vi "e.gate ASCII Read Value - CORE.vi"(8 "error in (no error)":errorcluster, 9 "Channel":i32, 11 "e.gate Configuration In":T1) -> (0 "error out":errorcluster, 2 "Value":dbl, 3 "e.gate Configuration Out":T1)   [LabVIEW 2016]
doc: "<B>AMC - Analytik & Messtechnik GmbH Chemnitz</B>\n\nLabVIEW Drivers for e.gate / e.pac series from Gantner Instruments\n\nThis VI reads a value specified by <B>Channel</B> from a device specified by <B>connection ID In</B>."
uses:
  e.gate Configuration.ctl
  e.gate Channel Data.ctl
  e.gate Data Type.ctl
  e.gate Protocol Type.ctl
  e.gate Module  Data.ctl
  e.gateHSP_DLLhandle.ctl
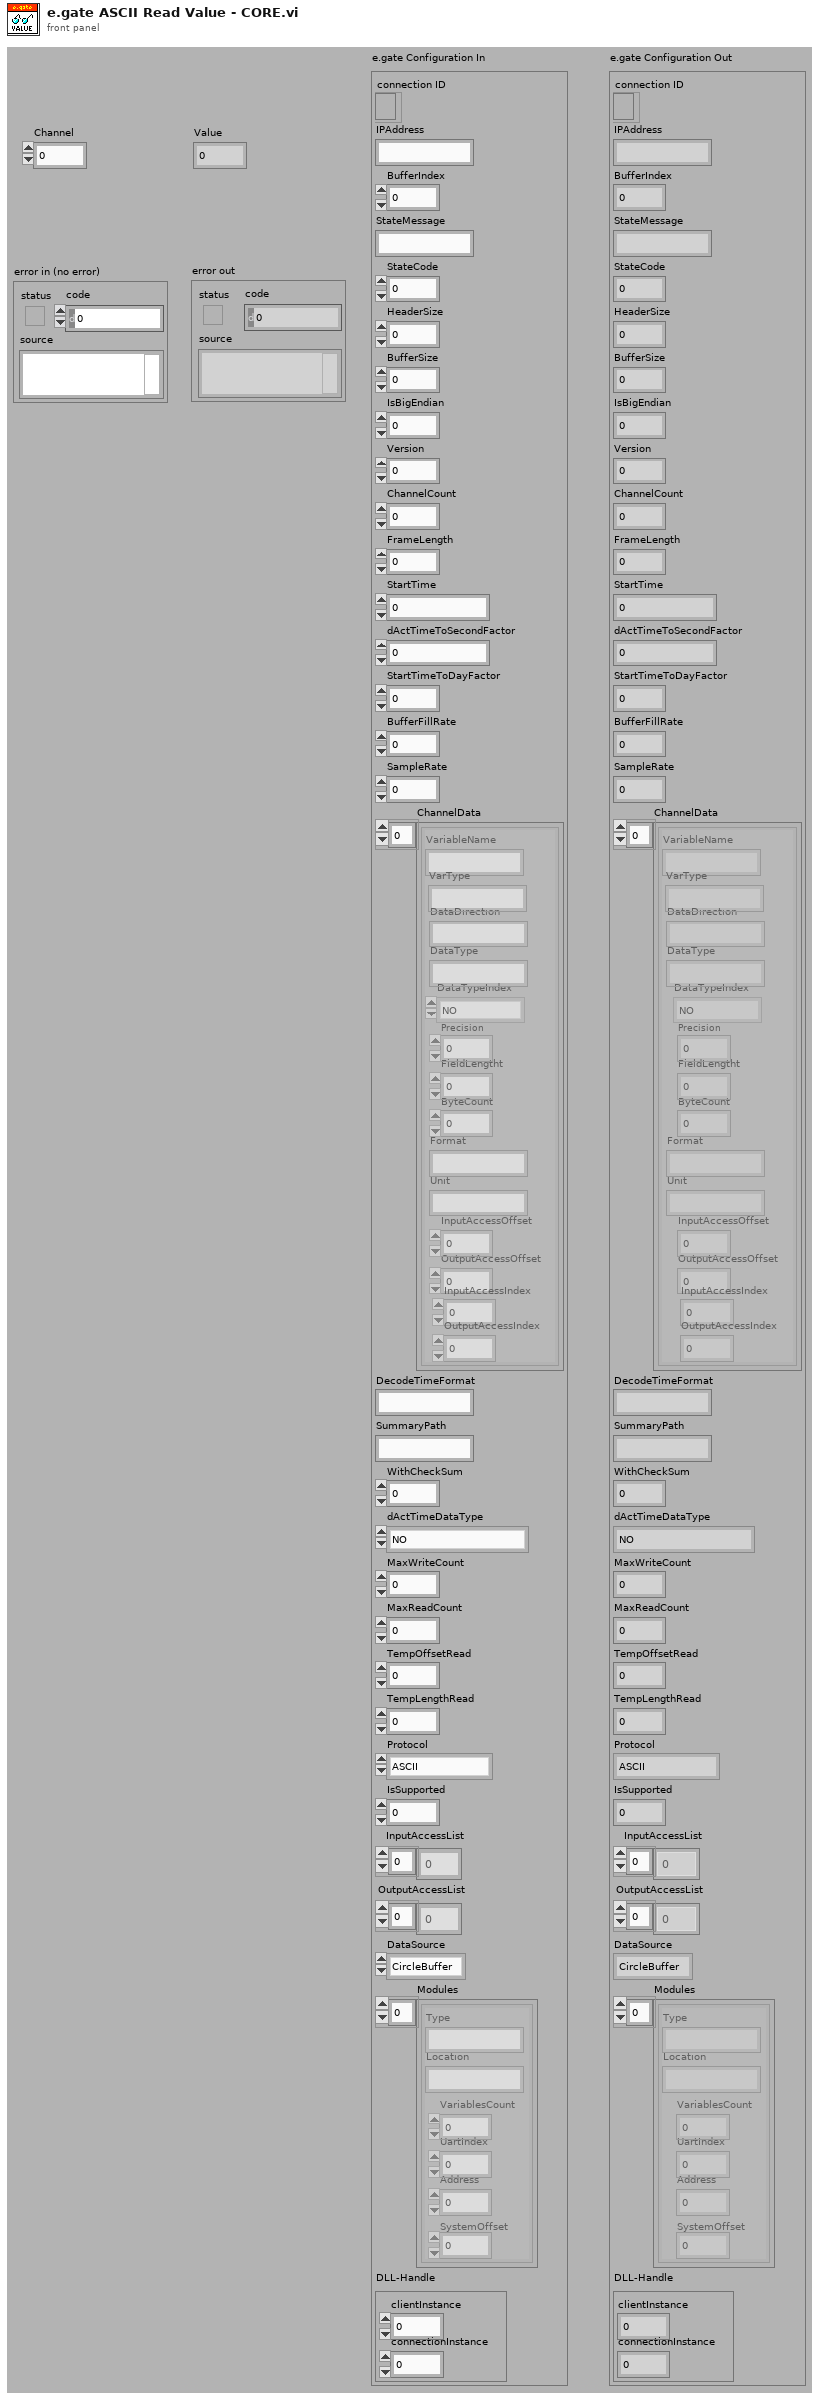
[diagram p1: front panel]
types:
  T1 = typedef "e.gate Configuration.ctl" = cluster{"connection ID":refnum<k5>, "IPAddress":string, "BufferIndex":i32, "StateMessage":string, "StateCode":i8, "HeaderSize":i32, "BufferSize":i32, "IsBigEndian":i32, "Version":i32, "ChannelCount":i32, "FrameLength":i32, "StartTime":dbl, "dActTimeToSecondFactor":dbl, "StartTimeToDayFactor":dbl, "BufferFillRate":dbl, "SampleRate":dbl, "ChannelData":T2[], "DecodeTimeFormat":string, "SummaryPath":string, "WithCheckSum":i32, "dActTimeDataType":T3, "MaxWriteCount":i32, "MaxReadCount":i32, "TempOffsetRead":i32, "TempLengthRead":i32, "Protocol":T4, "IsSupported":i32, "InputAccessList":i32[], "OutputAccessList":i32[], "DataSource":enum16{"CircleBuffer", "test.con Logger", "test.con Archive"}, "Modules":T5[], "DLL-Handle":T6}
  T2 = typedef "e.gate Channel Data.ctl" = cluster{"VariableName":string, "DataDirection":string, "DataType":string, "DataTypeIndex":T3, "Precision":i16, "FieldLengtht":i16, "ByteCount":i32, "Format":string, "Unit":string, "InputAccessOffset":i32, "OutputAccessOffset":i16, "InputAccessIndex":i16, "OutputAccessIndex":i16, "VarType":string}
  T3 = typedef "e.gate Data Type.ctl" = enum16{"NO", "BOOL", "SINT8", "USINT8", "SINT16", "USINT16", "SINT32", "USINT32", "FLOAT", "SET8", "SET16", "SET32", "DOUBLE", "SINT64", "USINT64", "SET64"}
  T4 = typedef "e.gate Protocol Type.ctl" = enum16{"ASCII", "HighspeedPort Online", "HighspeedPort Buffer", "eGateHighspeedPortDLL "}
  T5 = typedef "e.gate Module  Data.ctl" = cluster{"Type":string, "Location":string, "VariablesCount":i16, "UartIndex":i16, "Address":i16, "SystemOffset":i16}
  T6 = typedef "e.gateHSP_DLLhandle.ctl" = cluster{"clientInstance":i32, "connectionInstance":i32}
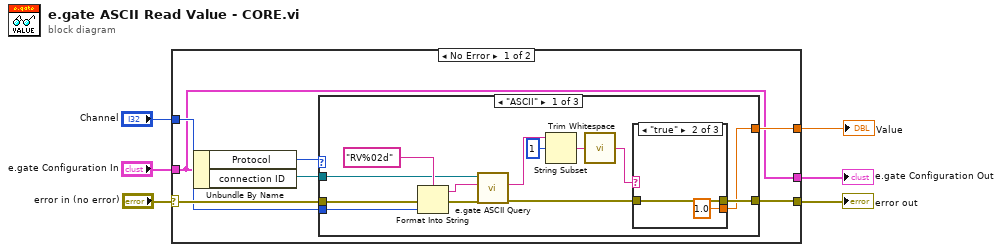
[diagram p0: block diagram]
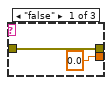
[diagram p2: hidden frame]
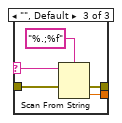
[diagram p3: hidden frame]
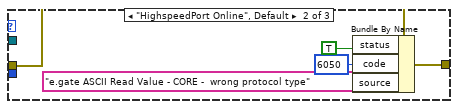
[diagram p4: hidden frame]
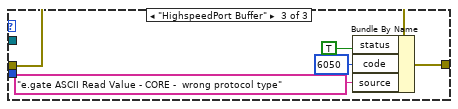
[diagram p5: hidden frame]
diagram:
  n1 = case shown="No Error" "error in (no error)" {
    selector: "error in (no error)" -> [w13 w47]
    tunnel: "e.gate Configuration In" -> [w9 w46]
    tunnel: "Channel" -> [w12 _]
    tunnel: [w9 w46] -> w3
    tunnel: [w11 w47] -> w2
    tunnel: [w10 _] -> w1
    frame No Error {
      n2 = Unbundle By Name(w9) -> ("Protocol"=w7:T4, "connection ID"=w8:refnum<k5>)
      n3 = case shown="\"ASCII\"" w7 {
        tunnel: w13 -> [w25 w40 w45]
        tunnel: w12 -> [w24 _ _]
        tunnel: [w15 w39 w44] -> w11
        tunnel: [w14 _ _] -> w10
        tunnel: w8 -> [w19 _ _]
        frame "ASCII" {
          n4 = Format Into String(format string="RV%02d", error in=w25, w24) -> (resulting string=w18:string, error out=w23:errorcluster)  [unwired: 1 in]
          n5 = call "e.gate ASCII Query.vi"("error in (no error)"=w23, "Command"=w18, "connection ID In"=w19) -> ("error out"=w16:errorcluster, "Response"=w20:string)  [unwired: 7 out]
          n6 = String Subset(string=w20, offset (0)=1) -> (substring=w21:string)  [unwired: 1 out]
          n7 = call <vilib>:"Trim Whitespace.vi"("string"=w21) -> ("trimmed string"=w17:string)  [unwired: 1 in]
          n8 = case shown="\"true\"" w17 {
            selector: w17 -> [_ _ w34]
            tunnel: w16 -> [w27 w30 w35]
            tunnel: [w27 w30 w32] -> w15
            tunnel: [0.0 1.0 w31] -> w14
            frame "false" {
            }
            frame "true" {
            }
            frame "", Default {
              n9 = Scan From String(format string="%.;%f", input string=w34, error in=w35) -> (error out=w32:errorcluster, output 1=w31:dbl)  [unwired: 1 in, 3 out]
            }
          }
        }
        frame "HighspeedPort Online", Default {
          n10 = Bundle By Name(cluster=w40, "status"=TRUE, "code"=6050, "source"="e.gate ASCII Read Value - CORE -  wrong protocol type") -> (w39:errorcluster)
        }
        frame "HighspeedPort Buffer" {
          n11 = Bundle By Name(cluster=w45, "status"=TRUE, "code"=6050, "source"="e.gate ASCII Read Value - CORE -  wrong protocol type") -> (w44:errorcluster)
        }
      }
    }
    frame Error {
    }
  }
  "error out" <- w2
  "e.gate Configuration Out" <- w3
  "Value" <- w1
